vi "AlazarGetNextBufferFloat.vi"(4 "error in (no error)":errorcluster, 5 "timeout_ms":u32, 6 "Buffer":sgl[](array[numeric]), 7 "Handle":u64) -> (0 "error out":errorcluster, 1 "Return Code":u32, 2 "Buffer":sgl[](array[numeric]), 3 "Handle":u64)   [LabVIEW 2018]
doc: "This function returns when the board has received sufficient trigger events to fill the buffer, or the timeout interval has elapsed. To use this function, AlazarBeforeAsyncRead must be called with the ADMA_ALLOC_BUFFERS flag."
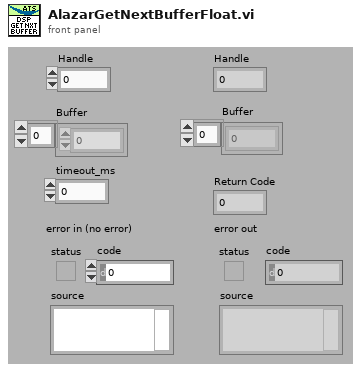
[diagram p1: front panel]
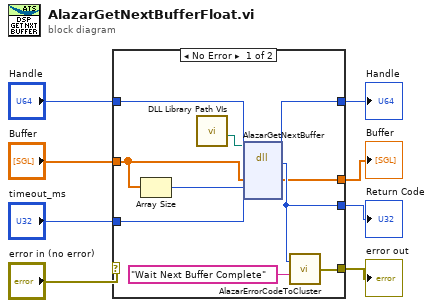
[diagram p0: block diagram]
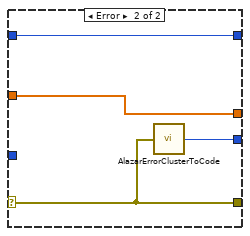
[diagram p2: hidden frame]
diagram:
  n1 = case shown="No Error" "error in (no error)" {
    selector: "error in (no error)" -> [_ w22]
    tunnel: [w15 w22] -> w7
    tunnel: [w17 w21] -> w6
    tunnel: "Handle" -> [w18 w20]
    tunnel: [w14 w20] -> w4
    tunnel: "Buffer" -> [w11 w19]
    tunnel: "timeout_ms" -> [w12 _]
    tunnel: [w13 w19] -> w1
    frame No Error {
      n2 = Array Size(array=w11) -> (size(s)=w10:i32)
      n3 = call "DLL Library Path VIs.vi"() -> ("Alazar"=w9:path)  [unwired: 9 in, 2 out]
      n4 = dll-call lib="C:/Project/SerialSectOCT - FFT GPU/SerialSectOCT/Labview Software/DLL/ATSApi.dll" fn="AlazarGetNextBuffer"(path in=w9, "handle"=w18, "buffer"=w11, "bytesToCopy"=w10, "timeout_ms"=w12) -> ("return type"=w17:i32, "handle"=w14:u64, "buffer"=w13:sgl[])  [unwired: 4 in, 2 out]
      n5 = call "AlazarErrorCodeToCluster.vi"("Message"="Wait Next Buffer Complete", "Error Code"=w17) -> ("error out"=w15:errorcluster)
    }
    frame Error {
      n6 = call "AlazarErrorClusterToCode.vi"("error in (no error)"=w22) -> ("Error Code"=w21:u32)
    }
  }
  "Handle" <- w4
  "error out" <- w7
  "Return Code" <- w6
  "Buffer" <- w1
